vi "(SubVI) Rotate judge.vi"(0 "x/y upper limit":dbl, 1 "x/y lower limit":dbl, 2 "Rotate time":i32=4, 3 "x position (delete y fit error)":dbl[](array[numeric]), 4 "y position (delete y fit error)":dbl[](array[numeric])) -> (5 "x = y?":bool)   [LabVIEW 2016]
uses:
  <vilib>/Analysis/coordinate.llb/2D Cartesian Coordinate Rotation (Array).vi
  <vilib>/Analysis/NI_AALPro.lvlib
  <vilib>/Analysis/NI_AALBase.lvlib
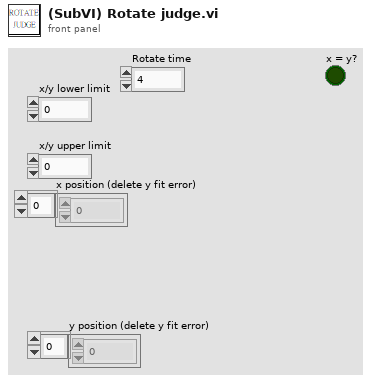
[diagram p1: front panel]
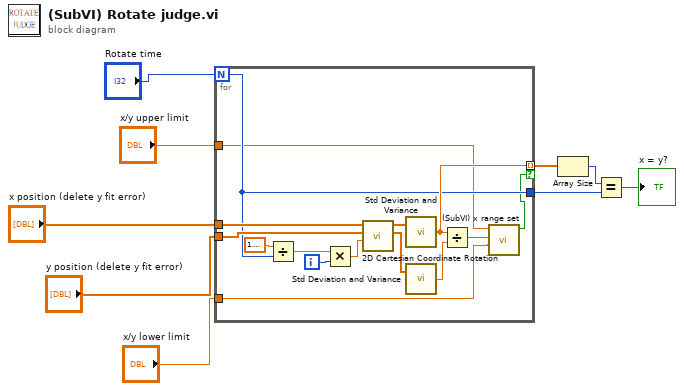
[diagram p0: block diagram]
diagram:
  n1 = for {
    N: "Rotate time" -> [w14]
    tunnel: "x position (delete y fit error)" -> [w24]
    tunnel: "y position (delete y fit error)" -> [w23]
    tunnel: "x/y upper limit" -> [w13]
    tunnel: "x/y lower limit" -> [w12]
    tunnel: [w15] -> w6 mode=indexing if=w10
    tunnel: [w14] -> w4
    i -> [w20]
    n2 = Divide(x=1.5707963267948966, y=w14) -> (x/y=w21:dbl)
    n3 = Multiply(x=w21, y=w20) -> (x*y=w19:dbl)
    n4 = call-poly <vilib>:"2D Cartesian Coordinate Rotation.vi"("theta"=w19, "Y"=w23, "X"=w24) -> ("Y Out"=w17:dbl[], "X Out"=w18:dbl[])  [unwired: 6 in, 1 out]
    n5 = call <vilib>:"Std Deviation and Variance.vi"("X"=w18) -> ("standard deviation"=w15:dbl)  [unwired: 1 in, 2 out]
    n6 = call <vilib>:"Std Deviation and Variance.vi"("X"=w17) -> ("standard deviation"=w16:dbl)  [unwired: 1 in, 2 out]
    n7 = Divide(x=w15, y=w16) -> (x/y=w11:dbl)
    n8 = call "(SubVI) x range set.vi"("lower limit"=w12, "x"=w11, "upper limit"=w13) -> ("Boolean"=w10:bool)  [unwired: 8 in]
  }
  n9 = Array Size(array=w6) -> (size(s)=w5:i32)
  n10 = Equal?(x=w5, y=w4) -> (x = y?=→"x = y?":bool)
